vi "run.vi"(8 "error in (no error)":errorcluster, 11 "HGF_SVMonitor in":refnum<class "HGF_SVMonitor.lvclass">) -> (0 "error out":errorcluster, 3 "HGF_SVMonitor out":refnum<class "HGF_SVMonitor.lvclass">)   [LabVIEW 2012, in "HGF_SV.lvlib" / "HGF_SVMonitor.lvclass"]
uses:
  HGF_SVMonitor.lvclass
  HGF_BaseClasses/HGF_NetworkVisitor/HGF_NetworkVisitor.lvclass
  HGF_BaseClasses/HGF_TriggeredEvent/HGF_TriggeredEvent.lvclass
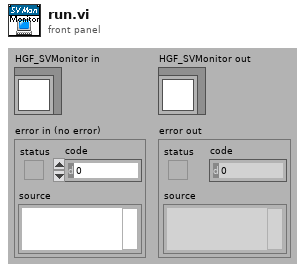
[diagram p1: front panel]
types:
  T1 = cluster{"registered Visitors":cluster{"HGF_NetworkVisitor":refnum<class "HGF_NetworkVisitor.lvclass">, "HGF_TriggeredEvent":refnum<class "HGF_TriggeredEvent.lvclass">}[], "last known data":variant, "Time Stamp":timestamp, "shared variable refnum in":refnum<k21>}[]
  T2 = cluster{"registered Visitors":cluster{"HGF_NetworkVisitor":refnum<class "HGF_NetworkVisitor.lvclass">, "HGF_TriggeredEvent":refnum<class "HGF_TriggeredEvent.lvclass">}[], "last known data":variant, "Time Stamp":timestamp, "shared variable refnum in":refnum<k21>}
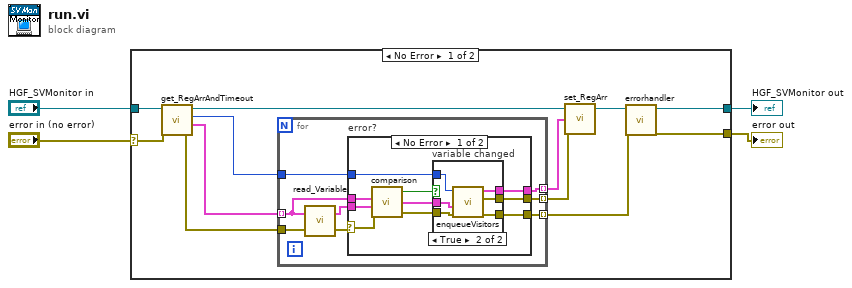
[diagram p0: block diagram]
diagram:
  n1 = case shown="No Error" "error in (no error)" {
    selector: "error in (no error)" -> [w12 w45]
    tunnel: [w5 w45] -> w3
    tunnel: [w6 w44] -> w1
    tunnel: "HGF_SVMonitor in" -> [w16 w44]
    frame No Error {
      n2 = call "get_RegArrAndTimeout.vi"("error in (no error)"=w12, "HGF_SVMonitor"=w16) -> ("error out"=w13:errorcluster, "Registration Array"=w14:T1, "timeout in ms(10)"=w15:i32, "HGF_SVMonitor"=w10:refnum<class "HGF_SVMonitor.lvclass">)  [unwired: 2 in]
      n3 = for {
        tunnel: w13 -> [w24]
        tunnel: w15 -> [w23]
        tunnel: w14 -> [w20] mode=indexing
        tunnel: [w19] -> w11 mode=indexing
        tunnel: [w18] -> w9 mode=indexing
        tunnel: [w17] -> w8 mode=indexing
        n4 = call "read_Variable.vi"("error in (no error)"=w24, "Variable Cluster"=w20) -> ("error out"=w22:errorcluster, "dup Variable Cluster"=w21:T2)
        n5 = case "error?" shown="No Error" w22 {
          selector: w22 -> [w31 w43]
          tunnel: w23 -> [w33 _]
          tunnel: w21 -> [w30 _]
          tunnel: w20 -> [w29 _]
          tunnel: [w27 w43] -> w19
          tunnel: [w26 _] -> w18
          tunnel: [w25 _] -> w17
          frame No Error {
            n6 = call "comparison.vi"("error in (no error)"=w31, "new Variable Cluster"=w30, "original Variable Cluster"=w29) -> ("error out"=w32:errorcluster, "Variable Cluster"=w28:T2, "change"=w34:bool)  [unwired: 1 in]
            n7 = case "variable changed" shown="True" w34 {
              tunnel: w33 -> [_ w41]
              tunnel: w32 -> [w35 w42]
              tunnel: [w35 w40] -> w27
              tunnel: w28 -> [w36 w39]
              tunnel: [w36 w38] -> w26
              tunnel: [w35 w37] -> w25
              frame False {
              }
              frame True {
                n8 = call "enqueueVisitors.vi"("error in (no error)"=w42, "Variable Cluster"=w39, "timeout in ms(10)"=w41) -> ("Event error out"=w37:errorcluster, "error out"=w40:errorcluster, "dup Variable Cluster"=w38:T2)  [unwired: 1 in, 1 out]
              }
            }
          }
          frame Error {
          }
        }
      }
      n9 = call "set_RegArr.vi"("Error Array"=w11, "Registration Array"=w9, "HGF_SVMonitor"=w10) -> ("HGF_SVMonitor"=w7:refnum<class "HGF_SVMonitor.lvclass">)  [unwired: 1 in]
      n10 = call-dynamic "errorhandler.vi"("HGF_SVMonitor in"=w7, "Error Array"=w8) -> ("HGF_SVMonitor out"=w6:refnum<class "HGF_SVMonitor.lvclass">, "error out"=w5:errorcluster)  [unwired: 16 out]
    }
    frame Error {
    }
  }
  "error out" <- w3
  "HGF_SVMonitor out" <- w1
